vi "CliDownload.vi"(0 "ref in":u64, 1 "Block Number":i32=1, 7 "Size":i32, 9 "data in":string, 11 "error in (no error)":errorcluster) -> (4 "ref out":u64, 6 "Result":i32, 15 "error out":errorcluster)   [LabVIEW 2010, in "Snap7.lvlib"]
uses:
  Snap7.lvlib
  windows/lv_snap7.dll
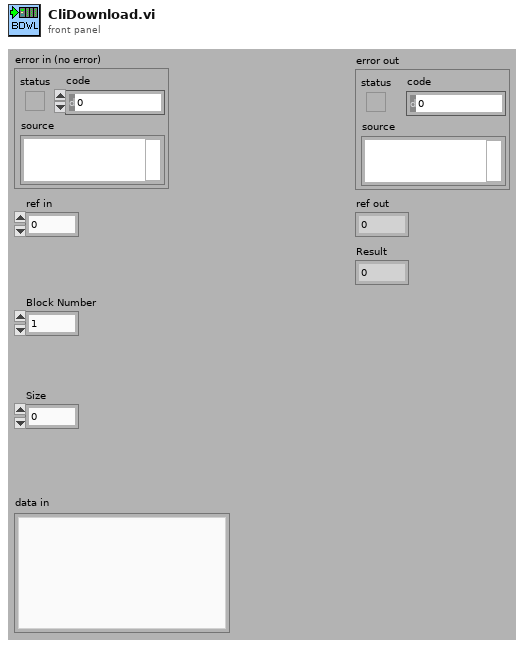
[diagram p1: front panel]
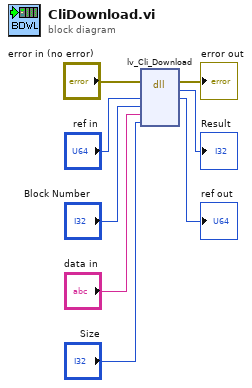
[diagram p0: block diagram]
diagram:
  n1 = dll-call lib="C:/snap7-src-1.0.0/LabVIEW/lib/windows/lv_snap7.dll" fn="lv_Cli_Download"(error in="error in (no error)", "Client"="ref in", "BlockNumber"="Block Number", "pUsrData"="data in", "Size"="Size") -> (error out=→"error out":errorcluster, "return type"=→"Result":i32, "Client"=→"ref out":u64)  [unwired: 5 in, 1 out]
